vi "Board State Terminal.vi"(11 "Board State":i32) -> (2 "Team":T1, 3 "Terminal?":bool)   [LabVIEW 2013]
uses:
  Typedef/Cell.ctl
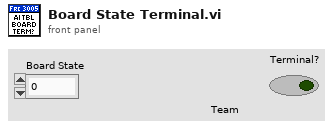
[diagram p1: front panel]
types:
  T1 = typedef "Cell.ctl" = enum16{"", "X", "O"}
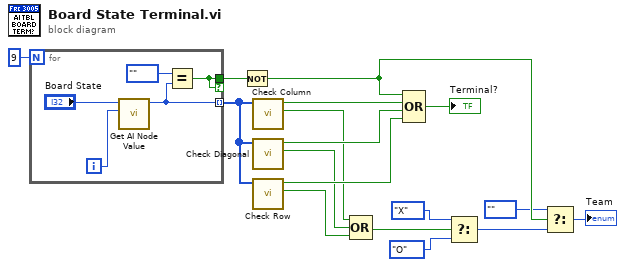
[diagram p0: block diagram]
diagram:
  n1 = for {
    N: 9 -> [_]
    tunnel: [w20] -> w17 mode=indexing
    tunnel: [w18] -> w13 if=w18
    i -> [w22]
    n2 = call "Get AI Node Value.vi"("Location"=w22, "Board State"="Board State") -> ("Value"=w20:T1)  [unwired: 9 in]
    n3 = Equal?(x=Cell."" ("Value"), y=w20) -> (x = y?=w18:bool)
  }
  n4 = Not(x=w13) -> (.not. x?=w4:bool)
  n5 = call "Check Column.vi"("Array"=w17) -> ("Team"=w10:bool, "Win?"=w16:bool)  [unwired: 9 in]
  n6 = call "Check Diagonal.vi"("Array"=w17) -> ("Team"=w9:bool, "Win?"=w15:bool)  [unwired: 9 in]
  n7 = call "Check Row.vi"("Array"=w17) -> ("Team"=w8:bool, "Win?"=w14:bool)  [unwired: 9 in]
  n8 = Compound Arithmetic op=OR(w10, w9, w8) -> (w7:bool)
  n9 = Compound Arithmetic op=OR(w4, w16, w15, w14) -> (→"Terminal?":bool)
  n10 = Select(t=Cell."X" ("Value"), s=w7, f=Cell."O" ("Value")) -> (s? t:f=w3:T1)
  n11 = Select(t=Cell."" ("Value"), s=w4, f=w3) -> (s? t:f=→"Team":T1)
